vi "GE 5565PIORC.DMA.Configure.vi"(7 "Transfer Direction":enum16{"Host to RFM", "RFM to Host"}(ring), 8 "error in (no error)":errorcluster, 10 "DMA Transfer Spec":T1 {"Block Descriptors"."descriptor params"."data ptr (lower)" format="%.0x"; "Block Descriptors"."descriptor params"."data ptr (upper)" format="%.0x"; "Block Descriptors"."descriptor params"."data size" format="%.0x"; "Block Descriptors"."descriptor params"."next descriptor ptr" format="%.0x"; "Block Descriptors"."descriptor size" format="%08x"; "Block Descriptors"."descriptor ptr (RFM)" format="%08x"; "Block Descriptors"."descriptor ptr (VISA)" format="%08x"; "RFM offset" format="%08x"}, 11 "GE 5565PIORC in":refnum<class "GE 5565PIORC.lvclass">) -> (0 "error out":errorcluster, 3 "GE 5565PIORC out":refnum<class "GE 5565PIORC.lvclass">)   [LabVIEW 2016, in "GE 5565PIORC.lvclass"]
doc: "Configures the required registers on the GE 5565PIORC to prepare for a DMA transfer as defined by <B>DMA Transfer Spec</B> and for the specified <B>Transfer Direction</B>."
uses:
  GE 5565PIORC.lvclass
  Typedefs/GE 5565PIORC.Typdef.DMA Transfer Spec.ctl
  Typedefs/GE 5565PIORC.Typdef.DMA Block Descriptor.ctl
  Typedefs/GE 5565PIORC.Typdef.DMA Block Descriptor Params.ctl
  GE 5565PIORC.lvclass/GE 5565PIORC.ctl
  Properties/Registers/GE 5565PIORC.Registers.Local Configuration.Read.vi
  Properties/Registers/GE 5565PIORC.Registers.Local Configuration.Read (U32).vi
  Properties/Registers/GE 5565PIORC.Registers.Local Configuration.Write.vi
  Properties/Registers/GE 5565PIORC.Registers.Local Configuration.Write (U32).vi
  Properties/Registers/Bit Manipulation.Set Bit.vi
  Properties/Registers/Bit Manipulation.Set Bit (U32).vi
  GE 5565PIORC.DMA.Scatter-Gather.Set Descriptor Params.vi
  Properties/Registers/GE 5565PIORC.Registers.Read.vi
  Properties/Registers/GE 5565PIORC.Registers.Read (U32).vi
  Properties/Registers/GE 5565PIORC.Registers.Write.vi
  Properties/Registers/GE 5565PIORC.Registers.Write (U32).vi
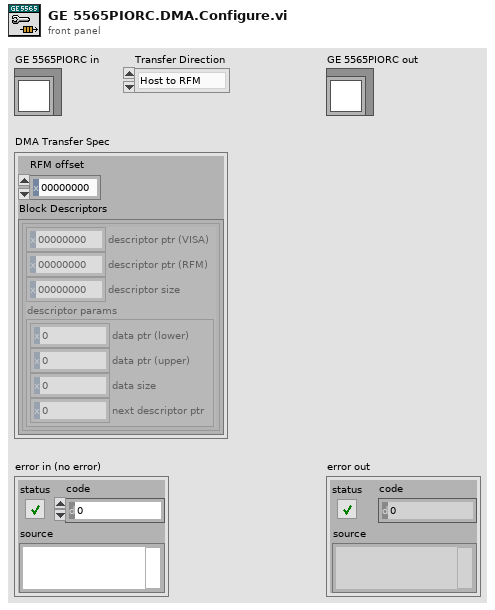
[diagram p1: front panel]
types:
  T1 = typedef "GE 5565PIORC.lvclass/GE 5565PIORC.Typdef.DMA Transfer Spec.ctl" = cluster{"RFM offset":u32, "Block Descriptors":T2[]}
  T2 = typedef "GE 5565PIORC.lvclass/GE 5565PIORC.Typdef.DMA Block Descriptor.ctl" = cluster{"descriptor ptr (VISA)":u32, "descriptor ptr (RFM)":u32, "descriptor size":u32, "descriptor params":T3}
  T3 = typedef "GE 5565PIORC.lvclass/GE 5565PIORC.Typdef.DMA Block Descriptor Params.ctl" = cluster{"data ptr (lower)":u32, "data ptr (upper)":u32, "data size":u32, "next descriptor ptr":u32}
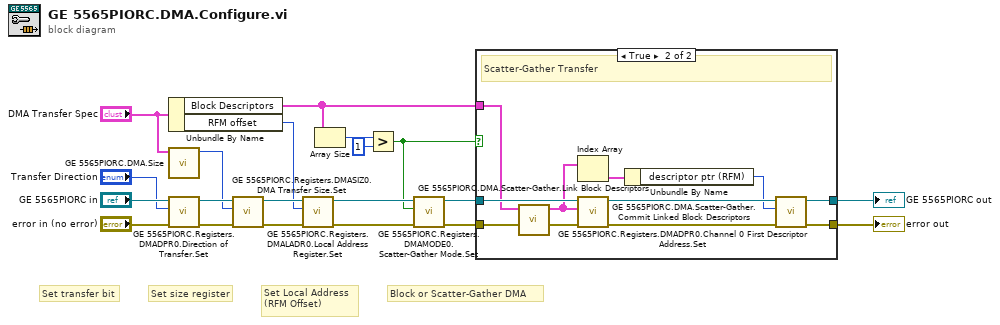
[diagram p0: block diagram]
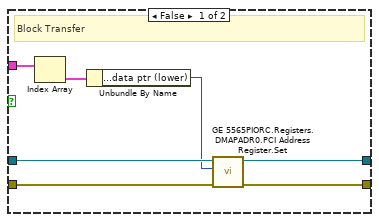
[diagram p2: hidden frame]
diagram:
  # "Block or Scatter-Gather DMA"
  # "Set Local Address (RFM Offset)"
  # "Set size register"
  # "Set transfer bit"
  n1 = Unbundle By Name("DMA Transfer Spec") -> ("Block Descriptors"=w1:T2[], "RFM offset"=w12:u32)
  n2 = call "GE 5565PIORC.DMA.Size.vi"("DMA Transfer Spec in"="DMA Transfer Spec") -> ("transfer size (bytes)"=w16:u32)  [unwired: 10 in]
  n3 = call "GE 5565PIORC.Registers.DMADPR0.Direction of Transfer.Set.vi"("error in (no error)"="error in (no error)", "Transfer Direction"="Transfer Direction", "GE 5565PIORC in"="GE 5565PIORC in") -> ("error out"=w17:errorcluster, "GE 5565PIORC out"=w18:refnum<class "GE 5565PIORC.lvclass">)  [unwired: 7 in]
  n4 = call "GE 5565PIORC.Registers.DMASIZ0.DMA Transfer Size.Set.vi"("error in (no error)"=w17, "DMA Transfer Size (Bytes)"=w16, "GE 5565PIORC in"=w18) -> ("error out"=w14:errorcluster, "GE 5565PIORC out"=w13:refnum<class "GE 5565PIORC.lvclass">)  [unwired: 7 in]
  n5 = call "GE 5565PIORC.Registers.DMALADR0.Local Address Register.Set.vi"("error in (no error)"=w14, "Local Address Register"=w12, "GE 5565PIORC in"=w13) -> ("error out"=w11:errorcluster, "GE 5565PIORC out"=w10:refnum<class "GE 5565PIORC.lvclass">)  [unwired: 7 in]
  n6 = Array Size(array=w1) -> (size(s)=w9:i32)
  n7 = Greater?(x=w9, y=1) -> (0:w7:bool)
  n8 = call "GE 5565PIORC.Registers.DMAMODE0.Scatter-Gather Mode.Set.vi"("error in (no error)"=w11, "Scatter-Gather Mode"=w7, "GE 5565PIORC in"=w10) -> ("error out"=w5:errorcluster, "GE 5565PIORC out"=w6:refnum<class "GE 5565PIORC.lvclass">)  [unwired: 7 in]
  n9 = case shown="True" w7 {
    tunnel: w1 -> [w26 w35]
    tunnel: w6 -> [w25 w36]
    tunnel: w5 -> [w24 w38]
    tunnel: [w22 w30] -> w4
    tunnel: [w21 w29] -> w3
    frame False {
      # "Block Transfer"
      n10 = Index Array(array=w26) -> (element=w27:T2)  [unwired: 1 in]
      n11 = Unbundle By Name(w27) -> ("descriptor params.data ptr (lower)"=w23:u32)
      n12 = call "GE 5565PIORC.Registers.DMAPADR0.PCI Address Register.Set.vi"("error in (no error)"=w24, "PCI Address Register"=w23, "GE 5565PIORC in"=w25) -> ("error out"=w21:errorcluster, "GE 5565PIORC out"=w22:refnum<class "GE 5565PIORC.lvclass">)  [unwired: 7 in]
    }
    frame True {
      # "Scatter-Gather Transfer"
      n13 = call "GE 5565PIORC.DMA.Scatter-Gather.Link Block Descriptors.vi"("error in (no error)"=w38, "Block Descriptors"=w35) -> ("error out"=w37:errorcluster, "Linked Block Descriptors"=w33:T2[])  [unwired: 8 in]
      n14 = Index Array(array=w33) -> (element=w34:T2)  [unwired: 1 in]
      n15 = call "GE 5565PIORC.DMA.Scatter-Gather.Commit Linked Block Descriptors.vi"("error in (no error)"=w37, "Linked Block Descriptors"=w33, "GE 5565PIORC in"=w36) -> ("error out"=w32:errorcluster, "GE 5565PIORC out"=w31:refnum<class "GE 5565PIORC.lvclass">)  [unwired: 7 in]
      n16 = Unbundle By Name(w34) -> ("descriptor ptr (RFM)"=w28:u32)
      n17 = call "GE 5565PIORC.Registers.DMADPR0.Channel 0 First Descriptor Address.Set.vi"("error in (no error)"=w32, "Channel 0 First Descriptor Address"=w28, "GE 5565PIORC in"=w31) -> ("error out"=w29:errorcluster, "GE 5565PIORC out"=w30:refnum<class "GE 5565PIORC.lvclass">)  [unwired: 7 in]
    }
  }
  "GE 5565PIORC out" <- w4
  "error out" <- w3
